vi "Create Class.vi"(8 "error in (no error)":errorcluster, 11 "Message Maker in":refnum<class "Abstract Message Rescripter.lvclass">) -> (0 "error out":errorcluster, 3 "Message Maker out":refnum<class "Abstract Message Rescripter.lvclass">)   [LabVIEW 2020, in "Message Rescripter.lvlib" / "Abstract Message Rescripter.lvclass"]
uses:
  Abstract Message Rescripter.lvclass
  <vilib>/Utility/EditLVLibs/Edit LVLibs.lvlib
  Message Rescripter.lvlib
  MessageMakerProvider/_Message Maker/Message Maker.lvlib
  MessageMakerProvider/_Message Maker/_Maker Classes/Message Scripter/Message Scripter.lvclass
  <vilib>/Utility/traverseref.llb/TRef TravTarget.ctl
  MessageMakerProvider/_Message Maker/_Maker Classes/Concrete Send Builder/Concrete Send Builder.lvclass
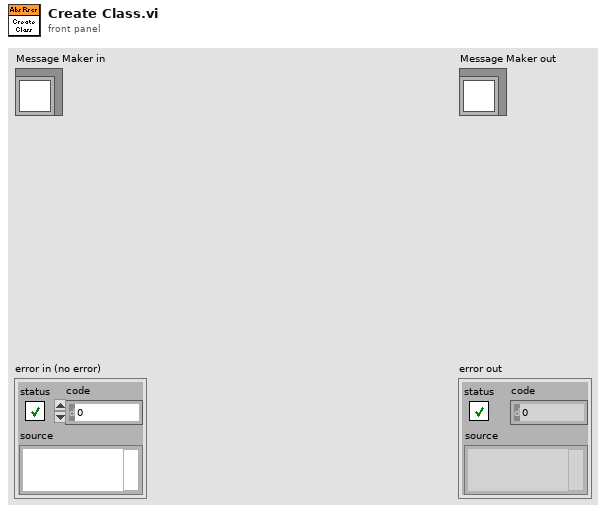
[diagram p1: front panel]
types:
  T1 = typedef "TRef TravTarget.ctl" = enum16{"FP", "BD", "Other"}
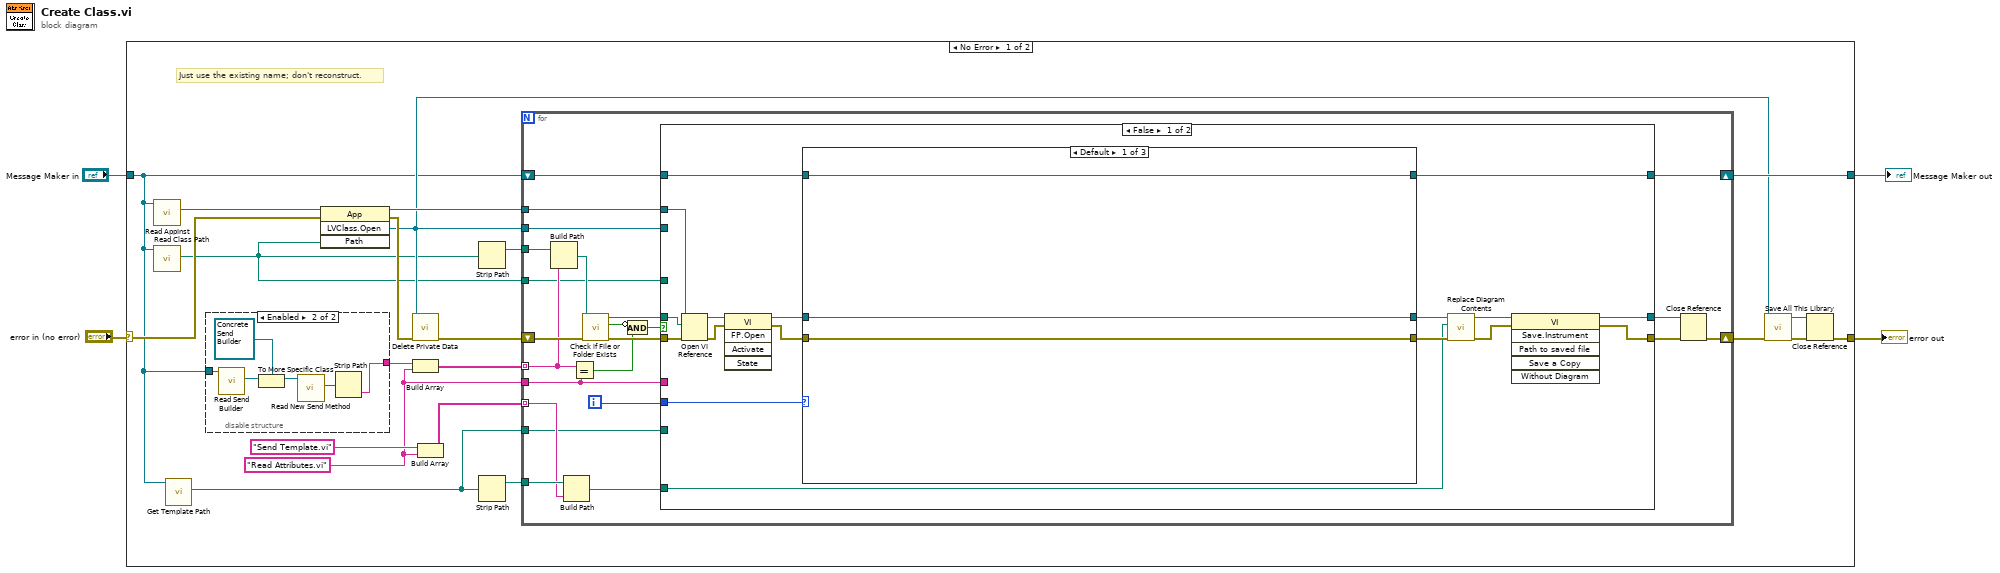
[diagram p0: block diagram]
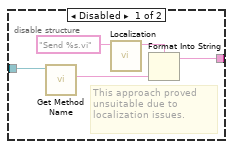
[diagram p2: hidden frame]
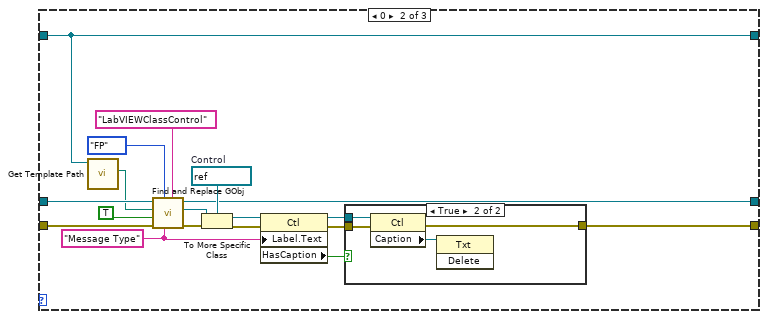
[diagram p3: hidden frame]
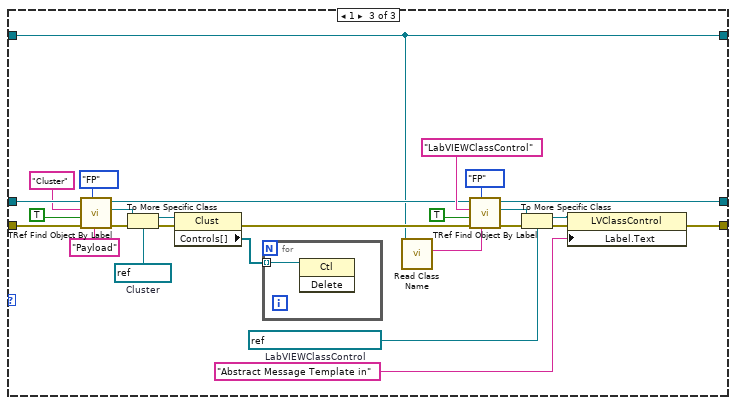
[diagram p5: hidden frame]
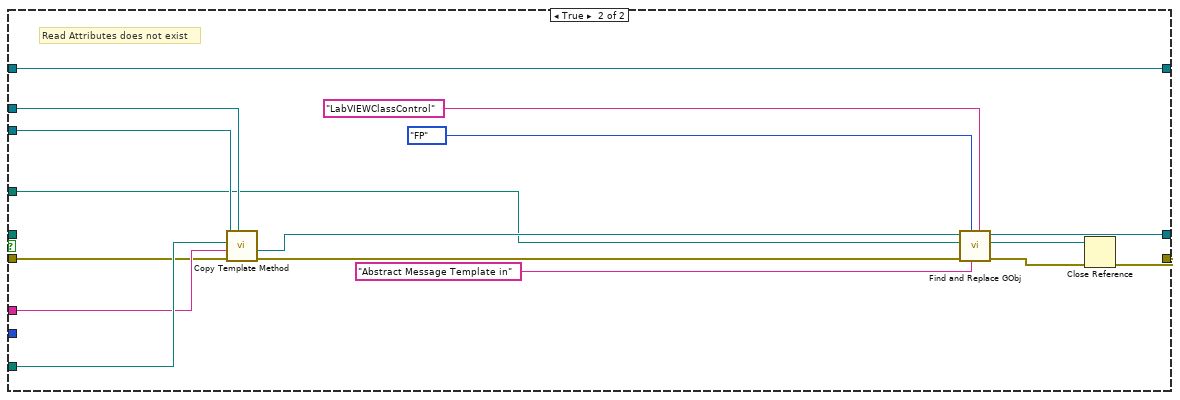
[diagram p6: hidden frame]
diagram:
  n1 = case shown="No Error" "error in (no error)" {
    selector: "error in (no error)" -> [w15 w148]
    tunnel: [w18 w148] -> w2
    tunnel: [w17 w147] -> w1
    tunnel: "Message Maker in" -> [w6 w147]
    frame No Error {
      w10 = "Read Attributes.vi" ("element")
      # "Just use the existing name; don't reconstruct."
      n2 = call "Read AppInst.vi"("Message Maker in"=w6) -> ("AppInst"=w13:refnum<vi>)  [unwired: 10 in]
      n3 = call "Read Class Path.vi"("Message Scripter in"=w6) -> ("Class Path"=w7:path)  [unwired: 10 in]
      n4 = call-dynamic "Get Template Path.vi"("Abstract Message Scripter in"=w6) -> ("Template Path"=w9:path)  [unwired: 10 in]
      n5 = disable-structure shown="Enabled" {
        disable-tunnel: [w28 w36] -> w20
        disable-tunnel: w6 -> [w27 w35]
        frame Disabled {
          # "This approach proved unsuitable due to localization issues."
          n6 = call-dynamic "Get Method Name.vi"("Message Maker in"=w27) -> ("Method Name"=w26:string)  [unwired: 10 in]
          n7 = call "Localization.vi"("Unlocalized"="Send %s.vi") -> ("Localized"=w29:string)  [unwired: 10 in]
          n8 = Format Into String(format string=w29, w26) -> (resulting string=w28:string)  [unwired: 2 in, 1 out]
        }
        frame Enabled {
          n9 = call-dynamic "Read Send Builder.vi"("Message Scripter in"=w35) -> ("Send Builder"=w34:refnum<class "Send Builder.lvclass">)  [unwired: 10 in]
          n10 = To More Specific Class(target class=refnum<class "Concrete Send Builder.lvclass"> refnum ("Concrete Send Builder in"), reference=w34) -> (specific class reference=w32:refnum<class "Concrete Send Builder.lvclass">)  [unwired: 1 in, 1 out]
          n11 = call-dynamic "Read New Send Method.vi"("Concrete Send Builder in"=w32) -> ("New Send Method"=w31:path)  [unwired: 10 in]
          n12 = Strip Path(path=w31) -> (name=w36:string)  [unwired: 1 out]
        }
      }
      n13 = invoke class="App" method="LVClass.Open"(reference=w13, error in=w15, "Path"=w7) -> (reference out=w24:refnum<vi>, error out=w16:errorcluster, "LVClass.Open"=w8:refnum<vi>)  [unwired: 1 in, 1 out]
      n14 = call "Delete Private Data.vi"("error in (no error)"=w16, "LVClassLibrary in"=w8) -> ("error out"=w25:errorcluster)  [unwired: 9 in]
      n15 = Build Array(w20, w10) -> (w22:string[])
      n16 = Build Array("Send Template.vi" ("Method"), w10) -> (w5:string[])
      n17 = Strip Path(path=w7) -> (stripped path=w12:path)  [unwired: 1 out]
      n18 = Strip Path(path=w9) -> (stripped path=w11:path)  [unwired: 1 out]
      n19 = for {
        shift-right: [w57] -> w23
        shift-left: w25 -> [w49]
        tunnel: w24 -> [w59]
        tunnel: w12 -> [w56]
        tunnel: w22 -> [w47] mode=indexing
        tunnel: w11 -> [w58]
        tunnel: w5 -> [w55] mode=indexing
        shift-right: [w53] -> w17
        shift-left: w6 -> [w54]
        tunnel: w10 -> [w45]
        tunnel: w9 -> [w46]
        tunnel: w8 -> [w44]
        tunnel: w7 -> [w37]
        i -> [w51]
        n20 = Build Path(base path=w56, name or relative path=w47) -> (appended path=w38:path)
        n21 = Build Path(base path=w58, name or relative path=w55) -> (appended path=w52:path)
        n22 = Equal?(x=w47, y=w45) -> (x = y?=w40:bool)
        n23 = call <vilib>:"Check if File or Folder Exists.vi"("error in (no error)"=w49, "path"=w38) -> ("error out"=w48:errorcluster, "file or folder exists?"=w41:bool, "dup path"=w50:path)  [unwired: 7 in]
        n24 = Compound Arithmetic op=AND(invert w41, w40) -> (w39:bool)
        n25 = case shown="False" w39 {
          tunnel: w59 -> [w76 w143]
          tunnel: w54 -> [w75 w141]
          tunnel: [w74 w141] -> w53
          tunnel: [w62 w135] -> w43
          tunnel: [w61 w133] -> w42
          tunnel: w52 -> [w71 _]
          tunnel: w51 -> [w66 _]
          tunnel: w50 -> [w65 _]
          tunnel: w48 -> [w64 w144]
          tunnel: w46 -> [_ w146]
          tunnel: w45 -> [_ w145]
          tunnel: w44 -> [_ w142]
          tunnel: w37 -> [_ w132]
          frame False {
            n26 = Open VI Reference(application reference (local)=w76, vi path=w65, error in (no error)=w64) -> (vi reference=w70:refnum<vi>, error out=w68:errorcluster)  [unwired: 3 in]
            n27 = invoke class="VI" method="FP.Open"(reference=w70, error in=w68) -> (reference out=w69:refnum<vi>, error out=w67:errorcluster)  [unwired: 3 in, 3 out]
            n28 = case shown="Default" w66 {
              tunnel: w69 -> [w78 w97 w121]
              tunnel: w67 -> [w77 w96 w124]
              tunnel: [w79 w95 w107] -> w74
              tunnel: w75 -> [w79 w95 w107]
              tunnel: [w78 w84 w109] -> w72
              tunnel: [w77 w81 w108] -> w73
              frame Default {
              }
              frame 0 {
                w88 = "Message Type" ("GObj Label")
                w90 = refnum<vi> refnum  # Control
                n29 = call-dynamic "Get Template Path.vi"("Abstract Message Scripter in"=w95) -> ("Template Path"=w94:path)  [unwired: 10 in]
                n30 = call "Find and Replace GObj.vi"("GObj Class Name"="LabVIEWClassControl", "GObj Label"=w88, "Traverse Target"=TRef_TravTarget."FP", "error in (no error)"=w96, "Case Insensitive Match? (F)"=TRUE, "Class Path"=w94, "vi reference in"=w97) -> ("error out"=w91:errorcluster, "Replace"=w83:refnum<vi>, "vi reference out"=w84:refnum<vi>)  [unwired: 2 in]
                n31 = To More Specific Class(target class=w90, reference=w83, error in=w91) -> (specific class reference=w89:refnum<vi>, error out=w82:errorcluster)
                n32 = property class="Ctl"(reference=w89, error in=w82, "Label.Text"=w88) -> (reference out=w86:refnum<vi>, error out=w85:errorcluster, "HasCaption"=w80:bool)
                n33 = case shown="True" w80 {
                  tunnel: w86 -> [_ w101]
                  tunnel: w85 -> [w98 w100]
                  tunnel: [w98 w99] -> w81
                  frame False {
                  }
                  frame True {
                    n34 = property class="Ctl"(reference=w101, error in=w100) -> (error out=w99:errorcluster, "Caption"=w102:refnum<vi>)  [unwired: 1 out]
                    n35 = invoke class="Txt" method="Delete"(reference=w102) -> ()  [unwired: 2 in, 3 out]
                  }
                }
              }
              frame 1 {
                w117 = refnum<vi> refnum  # LabVIEWClassControl
                w129 = refnum<vi> refnum  # Cluster
                n36 = call <vilib>:"TRef Find Object By Label.vi"("Label"="Payload" ("GObj Label"), "Traverse Target"=TRef_TravTarget."FP", "error in (no error)"=w124, "Case Insensitive Match? (F)"=TRUE, "Class Name"="Cluster" ("GObj Class Name"), "VI Ref"=w121) -> ("error out"=w123:errorcluster, "Found Obj Ref"=w122:refnum<vi>, "dup VI Ref"=w110:refnum<vi>)  [unwired: 2 in, 1 out]
                n37 = To More Specific Class(target class=w129, reference=w122, error in=w123) -> (specific class reference=w128:refnum<vi>, error out=w127:errorcluster)
                n38 = property class="Clust"(reference=w128, error in=w127) -> (error out=w111:errorcluster, "Controls[]"=w126:refnum<vi>[])  [unwired: 1 out]
                n39 = for {
                  tunnel: w126 -> [w130] mode=indexing
                  n40 = invoke class="Ctl" method="Delete"(reference=w130) -> ()  [unwired: 2 in, 3 out]
                }
                n41 = call "Read Class Name.vi"("Message Scripter in"=w107) -> ("Class Name"=w106:string)  [unwired: 10 in]
                n42 = call <vilib>:"TRef Find Object By Label.vi"("Label"=w106, "Traverse Target"=TRef_TravTarget."FP", "error in (no error)"=w111, "Case Insensitive Match? (F)"=TRUE, "Class Name"="LabVIEWClassControl", "VI Ref"=w110) -> ("error out"=w113:errorcluster, "Found Obj Ref"=w116:refnum<vi>, "dup VI Ref"=w109:refnum<vi>)  [unwired: 2 in, 1 out]
                n43 = To More Specific Class(target class=w117, reference=w116, error in=w113) -> (specific class reference=w118:refnum<vi>, error out=w115:errorcluster)
                n44 = property class="LVClassControl"(reference=w118, error in=w115, "Label.Text"="Abstract Message Template in" ("GObj Label")) -> (error out=w108:errorcluster)  [unwired: 1 out]
              }
            }
            n45 = call "Replace Diagram Contents.vi"("error in (no error)"=w73, "Template VI"=w71, "Target VI"=w72) -> ("error out"=w60:errorcluster, "dup Target VI"=w63:refnum<vi>)  [unwired: 7 in]
            n46 = invoke class="VI" method="Save.Instrument"(reference=w63, error in=w60) -> (reference out=w62:refnum<vi>, error out=w61:errorcluster)  [unwired: 4 in, 4 out]
          }
          frame True {
            # "Read Attributes does not exist"
            n47 = call "Copy Template Method.vi"("App Inst"=w143, "error in (no error)"=w144, "Method"=w145, "Template Class"=w146, "Message Class"=w142) -> ("error out"=w134:errorcluster, "Method Reference"=w138:refnum<vi>)  [unwired: 5 in]
            n48 = call "Find and Replace GObj.vi"("GObj Class Name"="LabVIEWClassControl" ("Class Name"), "GObj Label"="Abstract Message Template in", "Traverse Target"=TRef_TravTarget."FP", "error in (no error)"=w134, "Class Path"=w132, "vi reference in"=w138) -> ("error out"=w136:errorcluster, "Replace"=w137:refnum<vi>, "vi reference out"=w135:refnum<vi>)  [unwired: 3 in]
            n49 = Close Reference(reference=w137, error in (no error)=w136) -> (error out=w133:errorcluster)
          }
        }
        n50 = Close Reference(reference=w43, error in (no error)=w42) -> (error out=w57:errorcluster)
      }
      n51 = call <vilib>:"Save All This Library.vi"("error in (no error)"=w23, "Library in"=w8) -> ("error out"=w19:errorcluster, "Library out"=w14:refnum<vi>)  [unwired: 8 in]
      n52 = Close Reference(reference=w14, error in (no error)=w19) -> (error out=w18:errorcluster)
    }
    frame Error {
    }
  }
  "error out" <- w2
  "Message Maker out" <- w1
